vi "Command & Ack - Send Command.vi"(7 "Timeout (-1)":i32=-1, 8 "error in (no error)":errorcluster, 9 "Message Data":variant, 10 "Message":string, 11 "SV B-M (Host) in":refnum<class "SV B-M (Host).lvclass">) -> (0 "error out":errorcluster, 3 "SV B-M (Host) out":refnum<class "SV B-M (Host).lvclass">, 4 "Timeout?":bool)   [LabVIEW 2015, in "SV B-M (Host).lvclass"]
doc: "Send a command to the target."
uses:
  SV B-M (Host).lvclass
  Type Defs/Message Cluster.ctl
  SV B-M (Host).lvclass/SV B-M (Host).ctl
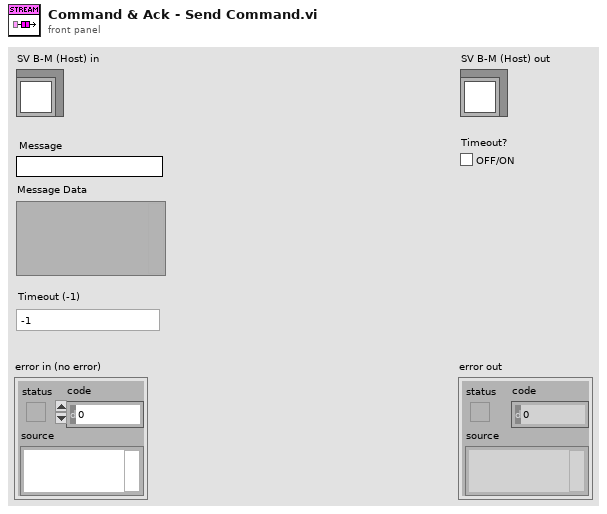
[diagram p1: front panel]
types:
  T1 = typedef "Message Cluster.ctl" = cluster{"Message":string, "Message Data":variant}
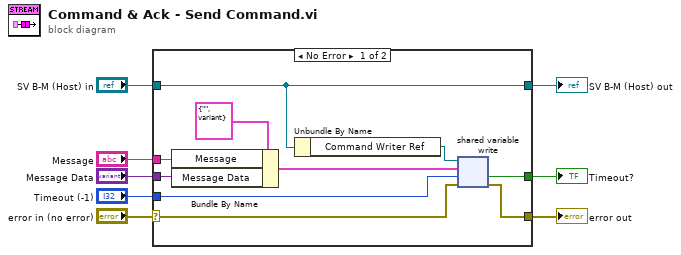
[diagram p0: block diagram]
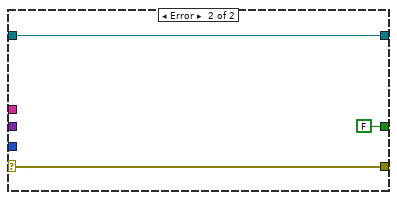
[diagram p2: hidden frame]
diagram:
  n1 = case shown="No Error" "error in (no error)" {
    selector: "error in (no error)" -> [w16 w21]
    tunnel: [w15 w21] -> w7
    tunnel: [w18 w20] -> w5
    tunnel: "SV B-M (Host) in" -> [w18 w20]
    tunnel: "Message" -> [w13 _]
    tunnel: "Message Data" -> [w12 _]
    tunnel: "Timeout (-1)" -> [w10 _]
    tunnel: [w9 FALSE] -> w1
    frame No Error {
      n2 = Bundle By Name(cluster=T1 {"Message"="", "Message Data"=variant} ("Message Cluster"), "Message"=w13, "Message Data"=w12) -> (w11:T1)
      n3 = Unbundle By Name(w18) -> ("Command Writer Ref"=w17:refnum<k21>)
      n4 = shared-variable-write(w17, w16, w11, w10) -> (w15:errorcluster, w9:bool)  [unwired: 1 out]
    }
    frame Error {
    }
  }
  "error out" <- w7
  "SV B-M (Host) out" <- w5
  "Timeout?" <- w1
